vi "Configure Gas Table Index.vi"(8 "error in (no error)":errorcluster, 10 "gas table index":u8, 11 "MKS MF1 in":refnum<class "PL MKS MF1 USB.lvclass">) -> (0 "error out":errorcluster, 3 "MKS MF1 out":refnum<class "PL MKS MF1 USB.lvclass">)   [LabVIEW 2015, in "PL MKS MF1 USB.lvclass"]
doc: "Configures gas table index."
uses:
  PL MKS MF1 USB.lvclass
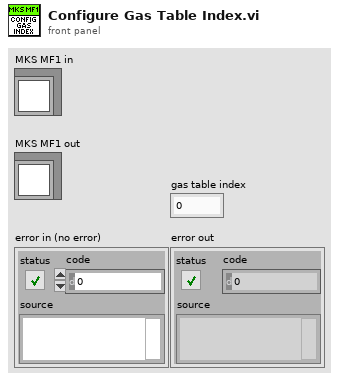
[diagram p1: front panel]
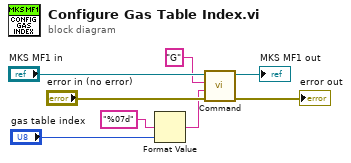
[diagram p0: block diagram]
diagram:
  n1 = Format Value(format string="%07d", value (0)="gas table index") -> (output string=w1:string)  [unwired: 1 in]
  n2 = call "Command.vi"("error in (no error)"="error in (no error)", "command value (no value)"=w1, "command"="G", "MKS MF1 in"="MKS MF1 in") -> ("error out"=→"error out":errorcluster, "MKS MF1 out"=→"MKS MF1 out":refnum<class "PL MKS MF1 USB.lvclass">)  [unwired: 4 in, 2 out]
